vi "h.SYSTEM.GetHlibVersion.vi"() -> (0 "h.Library Version":string)   [LabVIEW 2016, in "h.Library.lvlib"]
doc: "Use this VI to retrieve the h.Library.lvlib version number. This library provides all Hyperion LabView API VIs.\n\n<b>h.Library Version</b> - The h.Library version number"
uses:
  h.Library.lvlib
panel:
  # "Hyperion h.Library Version"
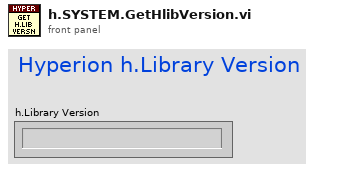
[diagram p1: front panel]
types:
  T1 = cluster{"Major":u16, "Minor":u16, "Fix":u16, "Build":u16}
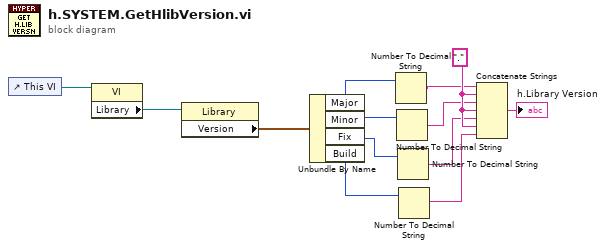
[diagram p0: block diagram]
diagram:
  w11 = "."
  n1 = control-ref of="This VI"() -> (w1:refnum<vi>)
  n2 = property class="VI"(reference=w1) -> ("Library"=w2:refnum<vi>)  [unwired: 1 in, 2 out]
  n3 = property class="Library"(reference=w2) -> ("Version"=w3:T1)  [unwired: 1 in, 2 out]
  n4 = Unbundle By Name(w3) -> ("Major"=w4:u16, "Minor"=w5:u16, "Fix"=w6:u16, "Build"=w7:u16)
  n5 = Number To Decimal String(number=w4) -> (decimal integer string=w8:string)  [unwired: 1 in]
  n6 = Number To Decimal String(number=w5) -> (decimal integer string=w9:string)  [unwired: 1 in]
  n7 = Number To Decimal String(number=w6) -> (decimal integer string=w10:string)  [unwired: 1 in]
  n8 = Number To Decimal String(number=w7) -> (decimal integer string=w12:string)  [unwired: 1 in]
  n9 = Concatenate Strings(w8, w11, w9, w11, w10, w11, w12) -> (→"h.Library Version":string)
